vi "quad gauss 1.vi"(3 "output control":T1, 4 "data":T2, 5 "X":dbl[](array[numeric]), 6 "a":dbl[](array[numeric])) -> (0 "error out":errorcluster, 1 "f'(X,a)":dbl[][](array[numeric]), 2 "f(X,a)":dbl[](array[numeric]))   [LabVIEW 2016]
doc: "This template is the starting point for creating a model function to be passed to the Nonlinear Curve Fit.vi."
uses:
  <vilib>/gmath/NumericalOptimization/objective function data.ctl
  <vilib>/gmath/NumericalOptimization/LM_output select.ctl
  <vilib>/gmath/NI_Gmath.lvlib
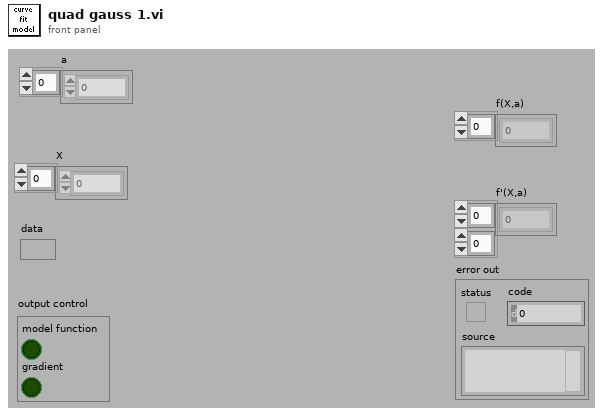
[diagram p1: front panel]
types:
  T1 = typedef "NI_Gmath.lvlib/LM_output select.ctl" = cluster{"model function":bool, "gradient":bool}
  T2 = typedef "NI_Gmath.lvlib/objective function data.ctl" = variant
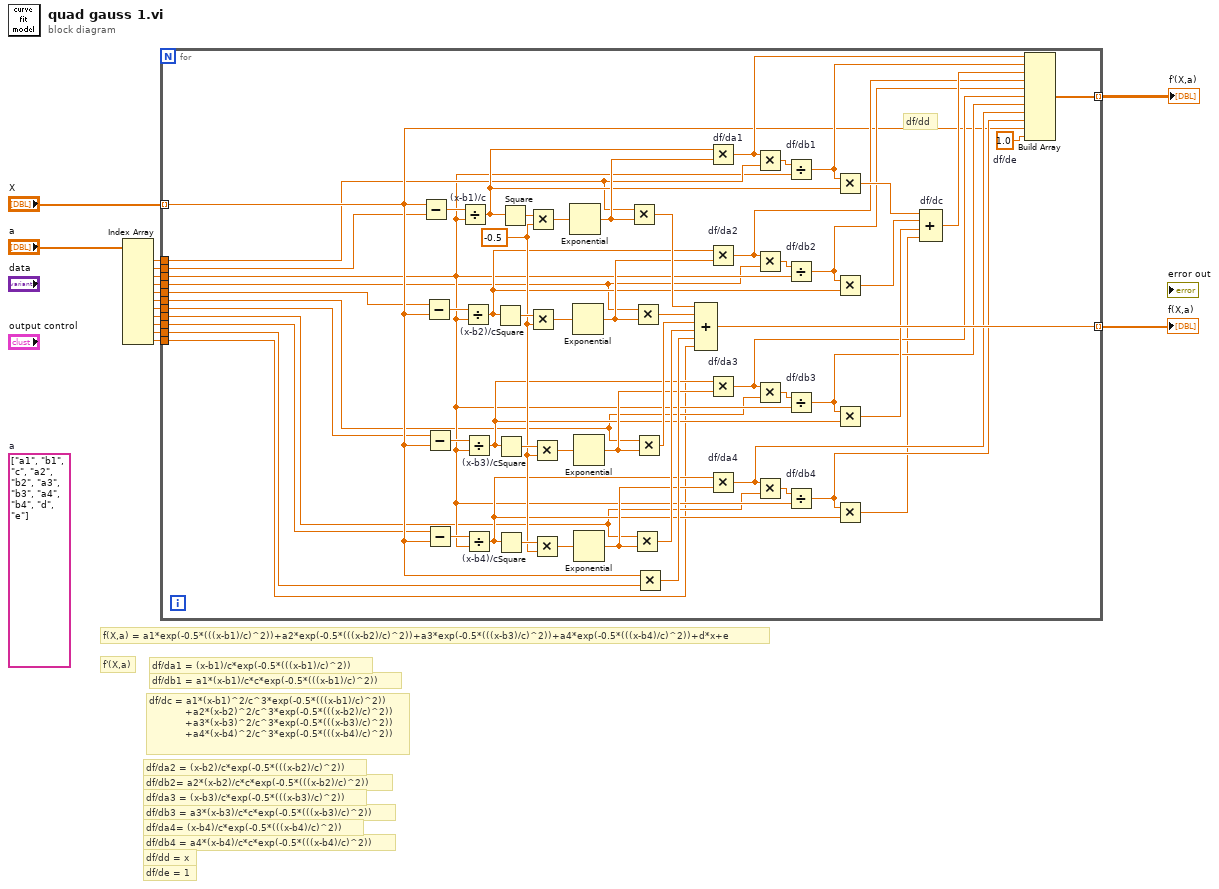
[diagram p0: block diagram]
diagram:
  (unwired) string[] ["a1", "b1", "c", "a2", "b2", "a3", "b3", "a4", "b4", "d", "e"]  # a
  # "f(X,a) = a1*exp(-0.5*(((x-b1)/c)^2))+a2*exp(-0.5*(((x-b2)/c)^2))+a3*exp(-0.5*(((x-b3)/c)^2))+a4*exp(-0.5*(((x-b4)/c)^2))+d*x+e"
  # "f'(X,a)"
  # "df/de = 1"
  # "df/dd = x"
  # "df/dc = a1*(x-b1)^2/c^3*exp(-0.5*(((x-b1)/c)^2))\n            +a2*(x-b2)^2/c^3*exp(-0.5*(((x-b2)/c)^2))\n            +a3*(x-b3)^2/c^3*exp(-0.5*(((x-b3)/c)^2))\n            +a4*(x-b4)^2/c^3*exp(-0.5*(((x-b4)/c)^2))"
  # "df/db4 = a4*(x-b4)/c*c*exp(-0.5*(((x-b4)/c)^2))"
  # "df/db3 = a3*(x-b3)/c*c*exp(-0.5*(((x-b3)/c)^2))"
  # "df/db2= a2*(x-b2)/c*c*exp(-0.5*(((x-b2)/c)^2))"
  # "df/db1 = a1*(x-b1)/c*c*exp(-0.5*(((x-b1)/c)^2))"
  # "df/da4= (x-b4)/c*exp(-0.5*(((x-b4)/c)^2))"
  # "df/da3 = (x-b3)/c*exp(-0.5*(((x-b3)/c)^2))"
  # "df/da2 = (x-b2)/c*exp(-0.5*(((x-b2)/c)^2))"
  # "df/da1 = (x-b1)/c*exp(-0.5*(((x-b1)/c)^2))"
  n1 = Index Array(array="a") -> (element #1=w11:dbl, element #2=w10:dbl, element #3=w9:dbl, element #4=w8:dbl, element #5=w7:dbl, element #6=w6:dbl, element #7=w5:dbl, element #8=w4:dbl, element #9=w3:dbl, element #10=w2:dbl, element #11=w1:dbl)  [unwired: 11 in]
  n2 = for {
    tunnel: "X" -> [w27] mode=indexing
    tunnel: [w60] -> w14 mode=indexing
    tunnel: [w52] -> w13 mode=indexing
    tunnel: w11 -> [w26]
    tunnel: w10 -> [w25]
    tunnel: w9 -> [w24]
    tunnel: w8 -> [w23]
    tunnel: w7 -> [w22]
    tunnel: w6 -> [w21]
    tunnel: w5 -> [w20]
    tunnel: w4 -> [w19]
    tunnel: w3 -> [w18]
    tunnel: w2 -> [w17]
    tunnel: w1 -> [w16]
    w28 = 1.0  # df/de
    w51 = -0.5 ("y")
    # "df/dd"
    n3 = Subtract(x=w27, y=w25) -> (x-y=w61:dbl)
    n4 = Subtract(x=w22, y=w27) -> (x-y=w66:dbl)
    n5 = Subtract(x=w20, y=w27) -> (x-y=w67:dbl)
    n6 = Subtract(x=w18, y=w27) -> (x-y=w72:dbl)
    n7 = Divide "(x-b1)/c"(x=w61, y=w24) -> (x/y=w45:dbl)
    n8 = Divide "(x-b2)/c"(x=w66, y=w24) -> (x/y=w44:dbl)
    n9 = Divide "(x-b3)/c"(x=w67, y=w24) -> (x/y=w38:dbl)
    n10 = Divide "(x-b4)/c"(x=w72, y=w24) -> (x/y=w32:dbl)
    n11 = Square(x=w44) -> (x^2=w65:dbl)
    n12 = Square(x=w38) -> (x^2=w68:dbl)
    n13 = Square(x=w32) -> (x^2=w71:dbl)
    n14 = Square(x=w45) -> (x^2=w62:dbl)
    n15 = Multiply(x=w62, y=w51) -> (x*y=w63:dbl)
    n16 = Multiply(x=w65, y=w51) -> (x*y=w64:dbl)
    n17 = Multiply(x=w68, y=w51) -> (x*y=w69:dbl)
    n18 = Multiply(x=w71, y=w51) -> (x*y=w70:dbl)
    n19 = Exponential(1:w63) -> (0:w54:dbl)
    n20 = Exponential(1:w64) -> (0:w46:dbl)
    n21 = Exponential(1:w69) -> (0:w39:dbl)
    n22 = Exponential(1:w70) -> (0:w33:dbl)
    n23 = Multiply(x=w26, y=w54) -> (x*y=w59:dbl)
    n24 = Multiply(x=w19, y=w33) -> (x*y=w56:dbl)
    n25 = Multiply(x=w23, y=w46) -> (x*y=w58:dbl)
    n26 = Multiply(x=w21, y=w39) -> (x*y=w57:dbl)
    n27 = Multiply(x=w27, y=w17) -> (x*y=w73:dbl)
    n28 = Compound Arithmetic op=ADD(w59, w58, w57, w56, w73, w16) -> (w60:dbl)
    n29 = Multiply "df/da1"(x=w45, y=w54) -> (x*y=w55:dbl)
    n30 = Multiply "df/da2"(x=w44, y=w46) -> (x*y=w42:dbl)
    n31 = Multiply "df/da3"(x=w38, y=w39) -> (x*y=w36:dbl)
    n32 = Multiply "df/da4"(x=w32, y=w33) -> (x*y=w31:dbl)
    n33 = Multiply(x=w55, y=w26) -> (x*y=w53:dbl)
    n34 = Multiply(x=w42, y=w23) -> (x*y=w47:dbl)
    n35 = Multiply(x=w36, y=w21) -> (x*y=w40:dbl)
    n36 = Multiply(x=w31, y=w19) -> (x*y=w34:dbl)
    n37 = Divide "df/db1"(x=w53, y=w24) -> (x/y=w50:dbl)
    n38 = Divide "df/db2"(x=w47, y=w24) -> (x/y=w41:dbl)
    n39 = Divide "df/db3"(x=w40, y=w24) -> (x/y=w35:dbl)
    n40 = Divide "df/db4"(x=w34, y=w24) -> (x/y=w30:dbl)
    n41 = Multiply(x=w50, y=w45) -> (x*y=w49:dbl)
    n42 = Multiply(x=w41, y=w44) -> (x*y=w43:dbl)
    n43 = Multiply(x=w35, y=w38) -> (x*y=w37:dbl)
    n44 = Multiply(x=w30, y=w32) -> (x*y=w29:dbl)
    n45 = Compound Arithmetic op=ADD "df/dc"(w49, w43, w37, w29) -> (w48:dbl)
    n46 = Build Array(w55, w50, w48, w42, w41, w36, w35, w31, w30, w27, w28) -> (w52:dbl[])
  }
  "f(X,a)" <- w14
  "f'(X,a)" <- w13
